vi "App_Auth_handler.vi"(8 "error in (no error)":errorcluster, 10 "Auth Time In":dbl, 11 "Path":path) -> (0 "error out":errorcluster, 2 "Auth Time Out":dbl, 3 "Codes":T1)   [LabVIEW 2016]
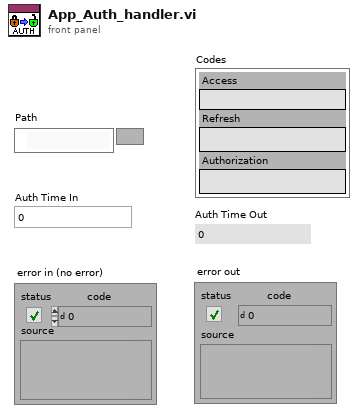
[diagram p1: front panel]
types:
  T1 = cluster{"Access":string, "Refresh":string, "Authorization":string}
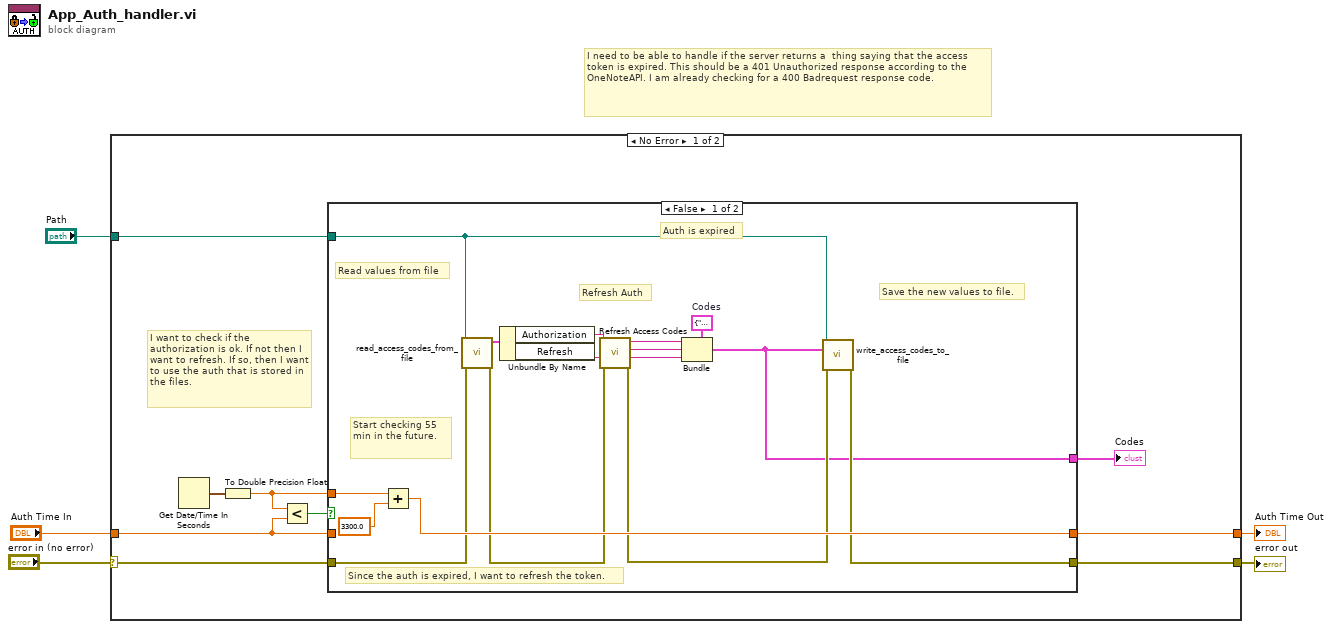
[diagram p0: block diagram]
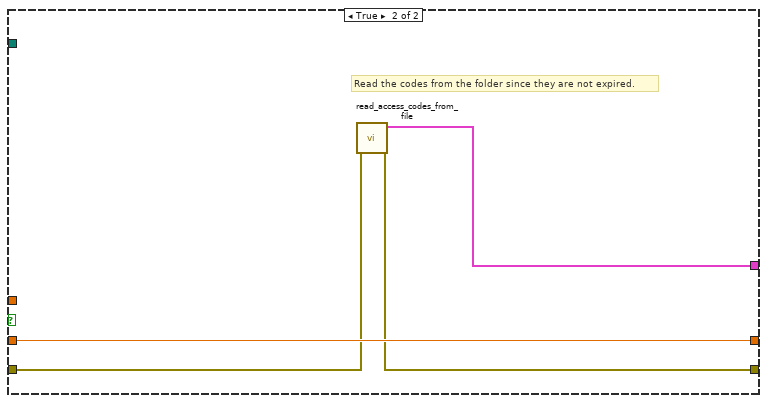
[diagram p2: hidden frame]
diagram:
  # "I need to be able to handle if the server returns a  thing saying that the access token is expired. This should be a 401 Unauthorized response according to the OneNoteAPI. I am already checking for a 400 Badrequest response code."
  n1 = case shown="No Error" "error in (no error)" {
    selector: "error in (no error)" -> [w11 w36]
    tunnel: [w7 w36] -> w4
    tunnel: "Auth Time In" -> [w10 w35]
    tunnel: [w9 w35] -> w2
    tunnel: "Path" -> [w8 _]
    frame No Error {
      # "I want to check if the authorization is ok. If not then I want to refresh. If so, then I want to use the auth that is stored in the files."
      n2 = Get Date/Time In Seconds() -> (seconds since 1Jan1904=w14:timestamp)
      n3 = To Double Precision Float(number=w14) -> (double precision float=w12:dbl)
      n4 = Less?(x=w12, y=w10) -> (x < y?=w13:bool)
      n5 = case shown="False" w13 {
        tunnel: w10 -> [_ w34]
        tunnel: w12 -> [w30 _]
        tunnel: [w28 w34] -> w9
        tunnel: w11 -> [w25 w31]
        tunnel: [w15 w32] -> w6
        tunnel: w8 -> [w18 _]
        tunnel: [w16 w33] -> w7
        frame False {
          w27 = T1 {"Access"="", "Refresh"="", "Authorization"=""}  # Codes
          # "Start checking 55 min in the future."
          # "Refresh Auth"
          # "Read values from file"
          # "Save the new values to file."
          # "Auth is expired"
          # "Since the auth is expired, I want to refresh the token."
          n6 = Add(x=w30, y=3300.0) -> (x+y=w28:dbl)
          n7 = call "read_access_codes_from_file.vi"("error in (no error)"=w25, "Path"=w18) -> ("error out"=w24:errorcluster, "Codes"=w26:T1)  [unwired: 8 in]
          n8 = Unbundle By Name(w26) -> ("Authorization"=w22:string, "Refresh"=w23:string)
          n9 = call "Refresh Access Codes.vi"("error in"=w24, "Refresh Token In"=w23, "Authorization Code In"=w22) -> ("error out"=w17:errorcluster, "Refresh Token Out"=w19:string, "Access Token Out"=w20:string, "Auth Code Out"=w21:string)  [unwired: 5 in]
          n10 = Bundle(cluster=w27, "Access"=w21, "Refresh"=w20, "Authorization"=w19) -> (w15:T1)
          n11 = call "write_access_codes_to_file.vi"("error in (no error)"=w17, "Cluster"=w15, "Path"=w18) -> ("error out"=w16:errorcluster)  [unwired: 8 in]
        }
        frame True {
          # "Read the codes from the folder since they are not expired."
          n12 = call "read_access_codes_from_file.vi"("error in (no error)"=w31) -> ("error out"=w33:errorcluster, "Codes"=w32:T1)  [unwired: 9 in]
        }
      }
      "Codes" <- w6
    }
    frame Error {
    }
  }
  "error out" <- w4
  "Auth Time Out" <- w2
